vi "PS Setup-hybrid.vi"(0 "vi reference":refnum<vi>) -> (4 "dup VI reference":refnum<vi>, 6 "Units":enum32{"tesla", "kAmps"}(radio) caption="tesla            kAmps", 7 "error out":errorcluster)   [LabVIEW 2020]
uses:
  PS Comm Globals.vi
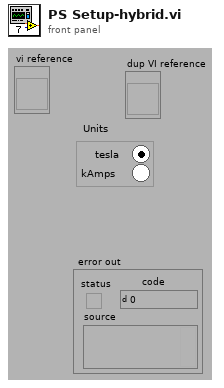
[diagram p1: front panel]
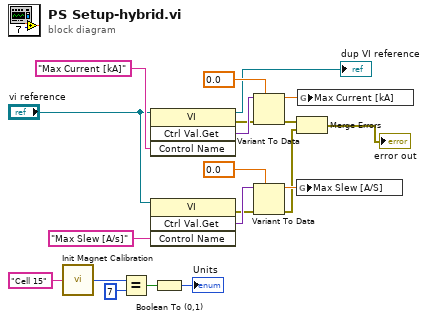
[diagram p0: block diagram]
diagram:
  n1 = call "Init Magnet Calibration.vi"("Magnet Id"="Cell 15") -> ("Error Code"=w19:i32)  [unwired: 2 out]
  n2 = Equal?(x=w19, y=7) -> (x = y?=w17:bool)
  n3 = invoke class="VI" method="Ctrl Val.Get"(reference="vi reference", "Control Name"="Max Current [kA]") -> (reference out=→"dup VI reference":refnum<vi>, error out=w7:errorcluster, "Get Control Value Variant"=w16:variant)  [unwired: 2 in, 1 out]
  n4 = invoke class="VI" method="Ctrl Val.Get"(reference="vi reference", "Control Name"="Max Slew [A/s]") -> (error out=w4:errorcluster, "Get Control Value Variant"=w8:variant)  [unwired: 2 in, 2 out]
  n5 = Boolean To (0,1)(Boolean=w17) -> (0, 1=→"Units":i16)
  n6 = Variant To Data(error in=w7, type=0.0 ("Current [KA]"), Variant=w16) -> (data=w13:dbl, error out=w6:errorcluster)
  n7 = Variant To Data(error in=w4, type=0.0 ("Current [KA]"), Variant=w8) -> (data=w11:dbl, error out=w5:errorcluster)
  n8 = Merge Errors(w6, w5) -> (→"error out":errorcluster)
  n9 = global write "PS Comm Globals.vi" "Max Slew [A/S]"(w11) -> ()
  n10 = global write "PS Comm Globals.vi" "Max Current [kA]"(w13) -> ()
